vi "Broadcast Response.vi"(8 "error in (no error)":errorcluster, 9 "Acquired Result.lvclass":refnum<class "Acquired Result.lvclass">, 10 "Topic":string, 11 "Measure Object in":refnum<class "PID Controller.lvclass">) -> (0 "error out":errorcluster, 3 "Measure Object out":refnum<class "PID Controller.lvclass">)   [LabVIEW 2019, in "PID Controller.lvclass"]
uses:
  PID Controller.lvclass
  NHMFL_Core/Libraries/Instruments/Results/Acquired Result/Acquired Result.lvclass
  <vilib>/addons/control/pid/pid.llb/PID (DBL).vi
  <vilib>/addons/control/pid/NI_PID_pid.lvlib
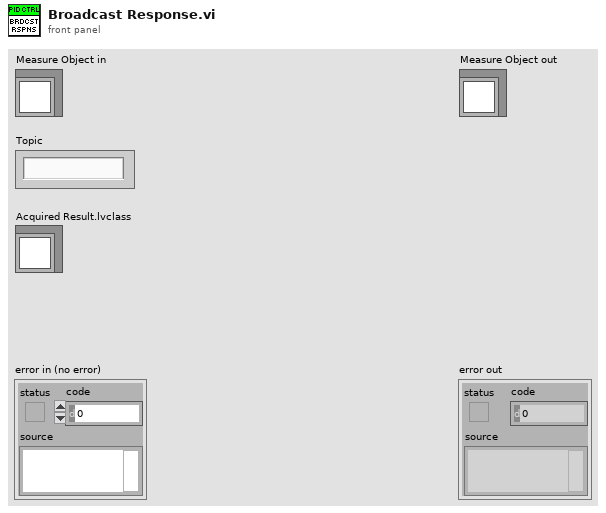
[diagram p1: front panel]
types:
  T1 = typedef "PID Controller Configuration.ctl" = cluster{"P":dbl, "I":dbl, "D":dbl, "Set point":dbl, "Input instrument":string, "Output instrument":string}
  T2 = cluster{"proportional gain (Kc)":dbl, "integral time (Ti, min)":dbl, "derivative time (Td, min)":dbl}
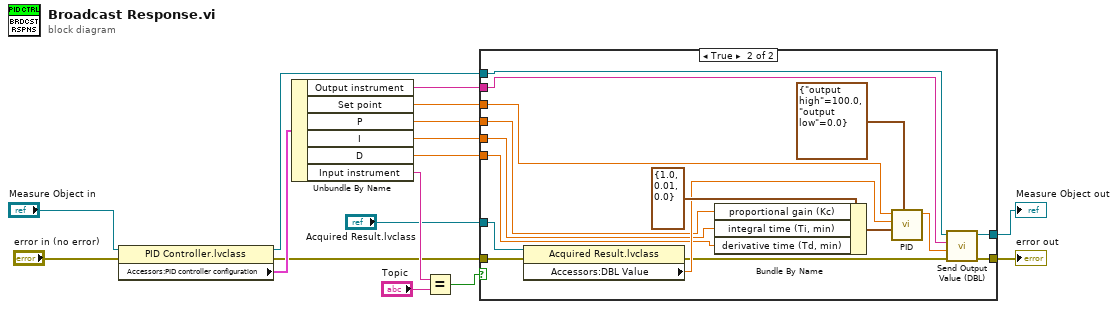
[diagram p0: block diagram]
diagram:
  n1 = property class="PID Controller.lvclass"(reference="Measure Object in", error in="error in (no error)") -> (reference out=w16:refnum<class "PID Controller.lvclass">, error out=w9:errorcluster, "Accessors:PID controller configuration"=w13:T1)
  n2 = Unbundle By Name(w13) -> ("Output instrument"=w1:string, "Set point"=w7:dbl, "P"=w6:dbl, "I"=w5:dbl, "D"=w4:dbl, "Input instrument"=w14:string)
  n3 = Equal?(x=w14, y="Topic") -> (x = y?=w15:bool)
  n4 = case shown="True" w15 {
    tunnel: w16 -> [w18 w24]
    tunnel: [w18 w23] -> w2
    tunnel: w9 -> [w17 w31]
    tunnel: "Acquired Result.lvclass" -> [_ w32]
    tunnel: w7 -> [_ w30]
    tunnel: w6 -> [_ w28]
    tunnel: w5 -> [_ w27]
    tunnel: w4 -> [_ w26]
    tunnel: [w17 w21] -> w3
    tunnel: w1 -> [_ w22]
    frame False {
    }
    frame True {
      n5 = property class="Acquired Result.lvclass"(reference=w32, error in=w31) -> (error out=w25:errorcluster, "Accessors:DBL Value"=w29:dbl)  [unwired: 1 out]
      n6 = Bundle By Name(cluster=T2 {"proportional gain (Kc)"=1.0, "integral time (Ti, min)"=0.01, "derivative time (Td, min)"=0.0} ("PID gains"), "proportional gain (Kc)"=w28, "integral time (Ti, min)"=w27, "derivative time (Td, min)"=w26) -> (w33:T2)
      n7 = call-poly <vilib>:"PID.vi"("output range"=cluster{"output high":dbl, "output low":dbl} {"output high"=100.0, "output low"=0.0}, "PID gains"=w33, "process variable"=w29, "setpoint"=w30) -> ("output"=w19:dbl)  [unwired: 6 in, 1 out]
      n8 = call-dynamic "Send Output Value (DBL).vi"("error in (no error)"=w25, "DBL Value"=w19, "Name"=w22, "Template Module in"=w24) -> ("error out"=w21:errorcluster, "Template Module out"=w23:refnum<class "PID Controller.lvclass">)  [unwired: 6 in]
    }
  }
  "error out" <- w3
  "Measure Object out" <- w2
